vi "Setting Database.FunnelsUpdated.vi"(8 "error in (no error)":errorcluster, 10 "FunnelsUpdated":T1, 11 "Setting Database":refnum<class "Setting Database.lvclass">) -> (0 "error out":errorcluster, 3 "Setting Database out":refnum<class "Setting Database.lvclass">)   [LabVIEW 2019, in "Setting Database.lvclass"]
doc: "---------------------------------------------------------------\nJKI State Machine Objects™\nhttp://jki.net/state-machine-objects/\nCopyright (C) 2005-2015, JKI <info@jki.net>\nALL RIGHTS RESERVEDJKI State Machine Objects (SMO) 1.0.0.4\nJKI - JKI\nCopyright (c) 2015, JKI"
uses:
  Setting Database.lvclass
  Typedefs/PublicEvents--Setting Database.FunnelsUpdated.ctl
  Funnel Settings/Funnel Settings.lvclass
  Typedefs/PublicEvents--Setting Database.FunnelsUpdatedCheck.ctl
  Setting Database.lvclass/Setting Database.ctl
panel:
  # "For instructions on how to use the JKI State Machine Objects, examples and video tutorials, visit:\nhttp://jki.net/state-machine-objects/\n\nJKI State Machine Objects™\nhttp://jki.net/state-machine-objects/\nCopyright (C) 2005-2015, JKI <info@jki.net>\nALL RIGHTS RESERVED"
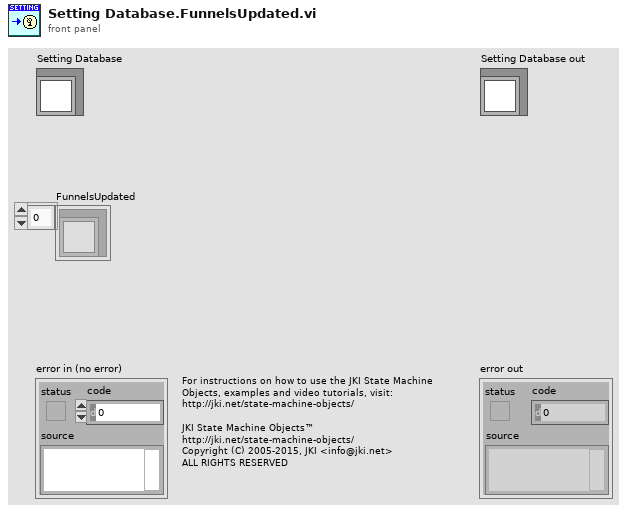
[diagram p1: front panel]
types:
  T1 = typedef "Setting Database.lvclass/PublicEvents--Setting Database.FunnelsUpdated.ctl" = refnum<class "Funnel Settings.lvclass">[]
  T2 = typedef "Setting Database.lvclass/PublicEvents--Setting Database.FunnelsUpdatedCheck.ctl" = cluster{"Read?":refnum<notifier>, "FunnelsUpdated":T1}
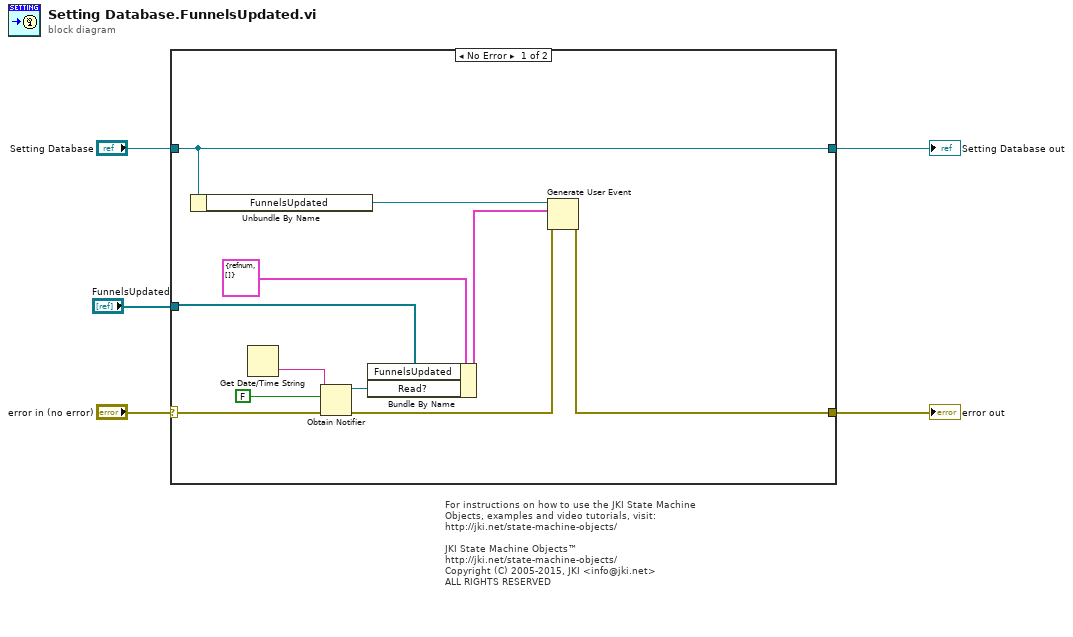
[diagram p0: block diagram]
diagram:
  # "For instructions on how to use the JKI State Machine Objects, examples and video tutorials, visit:\nhttp://jki.net/state-machine-objects/\n\nJKI State Machine Objects™\nhttp://jki.net/state-machine-objects/\nCopyright (C) 2005-2015, JKI <info@jki.net>\nALL RIGHTS RESERVED"
  n1 = case shown="No Error" "error in (no error)" {
    selector: "error in (no error)" -> [w11 w18]
    tunnel: [w15 w18] -> w4
    tunnel: [w14 w17] -> w5
    tunnel: "Setting Database" -> [w14 w17]
    tunnel: "FunnelsUpdated" -> [w6 _]
    frame No Error {
      n2 = Unbundle By Name(w14) -> ("FunnelsUpdated"=w16:refnum<user-event>)
      n3 = Get Date/Time String() -> (time string=w12:string)  [unwired: 3 in, 1 out]
      n4 = Obtain Notifier(name (unnamed)=w12, notification data type=FALSE, error in (no error)=w11) -> (notifier out=w8:refnum<notifier>, error out=w10:errorcluster)  [unwired: 1 in, 1 out]
      n5 = Bundle By Name(cluster=T2 {"Read?"=refnum, "FunnelsUpdated"=[]} ("FunnelsUpdated"), "FunnelsUpdated"=w6, "Read?"=w8) -> (w7:T2)
      n6 = Generate User Event(user event=w16, event data cluster=w7, error in=w10) -> (error out=w15:errorcluster)  [unwired: 1 in, 1 out]
    }
    frame Error {
    }
  }
  "error out" <- w4
  "Setting Database out" <- w5
